vi "IFS.vi"(0 "System no.":i32=1 min=1 step=1, 2 "Interface parameter":string[](array[string]), 3 "Parameter value":string[](array[string]), 4 "Password":string="100", 5 "error in":errorcluster) -> (19 "error out":errorcluster)   [LabVIEW 2020]
doc: "If Password is correct, the default parameter(s) for the interface are changed, but the current active parameters are not changed. Settings made with IFS are saved to EPROM and become active with the next startup/reboot. To change settings immediately (but temporarily) use IFC instead (if supported by your controller).\n\nE-709: Interface parameter can only be RSBAUD.\n\nC-887, F-206, M-8X0: Only for GCS syntax version = GCS 2.0 or higher (check with CSV?.vi. If CSV?.vi is not supported, syntax version is GCS 1.0)."
panel:
  # "If Password is correct, the default parameter(s) for the interface are changed, but the \ncurrent active parameters are not changed. Settings made with IFS are saved to EPROM \nand become active with the next startup/reboot. To change settings immediately (but \ntemporarily) use IFC instead (if supported by your controller)."
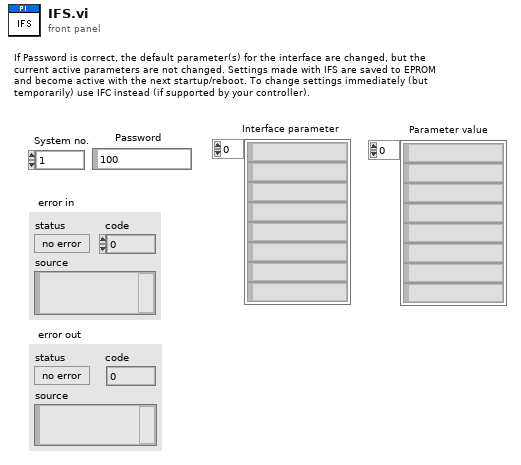
[diagram p1: front panel]
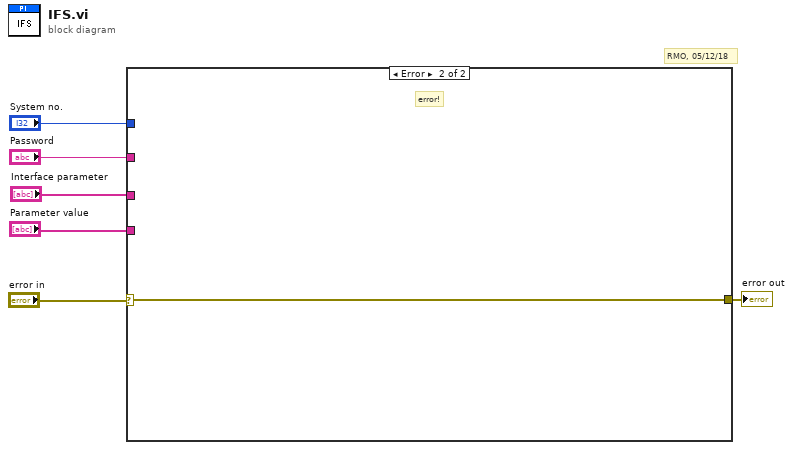
[diagram p0: block diagram]
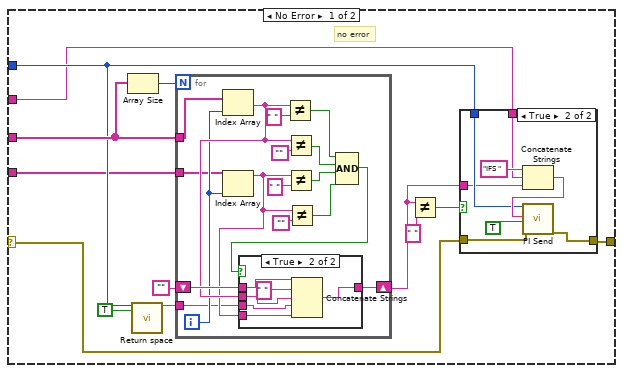
[diagram p2: hidden frame]
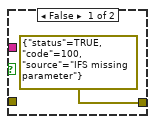
[diagram p3: hidden frame]
diagram:
  # "RMO, 05/12/18"
  n1 = case shown="Error" "error in" {
    selector: "error in" -> [w7 w53]
    tunnel: "Interface parameter" -> [w19 _]
    tunnel: [w10 w53] -> w5
    tunnel: "Parameter value" -> [w17 _]
    tunnel: "System no." -> [w18 _]
    tunnel: "Password" -> [w8 _]
    frame No Error {
      # "no error"
      n2 = Array Size(array=w19) -> (size(s)=w12:i32)
      n3 = call "Return space.vi"("System no."=w18, "With space?"=TRUE) -> ("String out"=w11:string)  [unwired: 17 out]
      n4 = for {
        N: w12 -> [_]
        tunnel: w19 -> [w34]
        shift-right: [w43] -> w14
        shift-left: "" -> [w44]
        tunnel: w17 -> [w32]
        tunnel: w11 -> [w29]
        i -> [w33]
        n5 = Index Array(array=w34, index=w33) -> (element=w42:string)
        n6 = Index Array(array=w32, index=w33) -> (element=w31:string)
        n7 = Not Equal?(x=w42, y=" ") -> (x != y?=w38:bool)
        n8 = Not Equal?(x=w42, y="") -> (x != y?=w37:bool)
        n9 = Not Equal?(x=w31, y=" ") -> (x != y?=w36:bool)
        n10 = Not Equal?(x=w31, y="") -> (x != y?=w35:bool)
        n11 = Compound Arithmetic op=AND(w38, w37, w36, w35) -> (w30:bool)
        n12 = case shown="True" w30 {
          tunnel: w44 -> [w46 w52]
          tunnel: w42 -> [_ w49]
          tunnel: [w46 w51] -> w43
          tunnel: w31 -> [_ w48]
          tunnel: w29 -> [_ w47]
          frame False {
          }
          frame True {
            n13 = Concatenate Strings(w52, " ", w49, w47, w48) -> (w51:string)
          }
        }
      }
      n14 = Not Equal?(x=w14, y=" ") -> (x != y?=w13:bool)
      n15 = case shown="True" w13 {
        tunnel: w14 -> [_ w21]
        tunnel: w7 -> [_ w25]
        tunnel: w18 -> [_ w24]
        tunnel: [errorcluster {"status"=TRUE, "code"=100, "source"="IFS missing parameter"} ("error out") w23] -> w10
        tunnel: w8 -> [_ w22]
        frame False {
        }
        frame True {
          n16 = Concatenate Strings("IFS ", w22, w21) -> (w26:string)
          n17 = call "PI Send.vi"("System no."=w24, "String to send"=w26, "Attach termination char.?"=TRUE ("Attach Linefeed?"), "error in"=w25) -> ("error out"=w23:errorcluster)  [unwired: 2 in, 13 out]
        }
      }
    }
    frame Error {
      # "error!"
    }
  }
  "error out" <- w5
